vi "Sweep_bias_voltage_GSM-20H10_TektronixMDO.vi"() -> ()   [LabVIEW 2016]
uses:
  <vilib>/Utility/file.llb/Write Delimited Spreadsheet (DBL).vi
panel:
  out "Running index":i32
  out "appended array":sgl[][](array[numeric])
  out "Waveform Graph":sgl[][](graph)
  in  "Number of Points (5)":u32=5
  in  "File Name":string="C:\\Users\\user01\\Desktop\\hsinyeh\\SNSPD_Data\\20230411\\2.5M_6.1K_10photons_0.68uW_"
  out "path":path
  in  "Input voltage":dbl[](array[numeric])
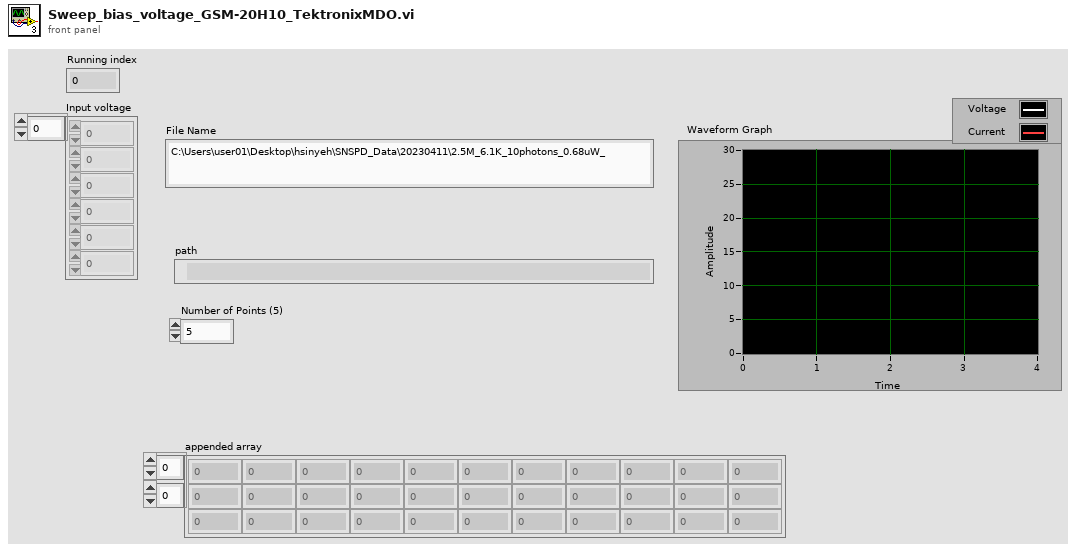
[diagram p1: front panel]
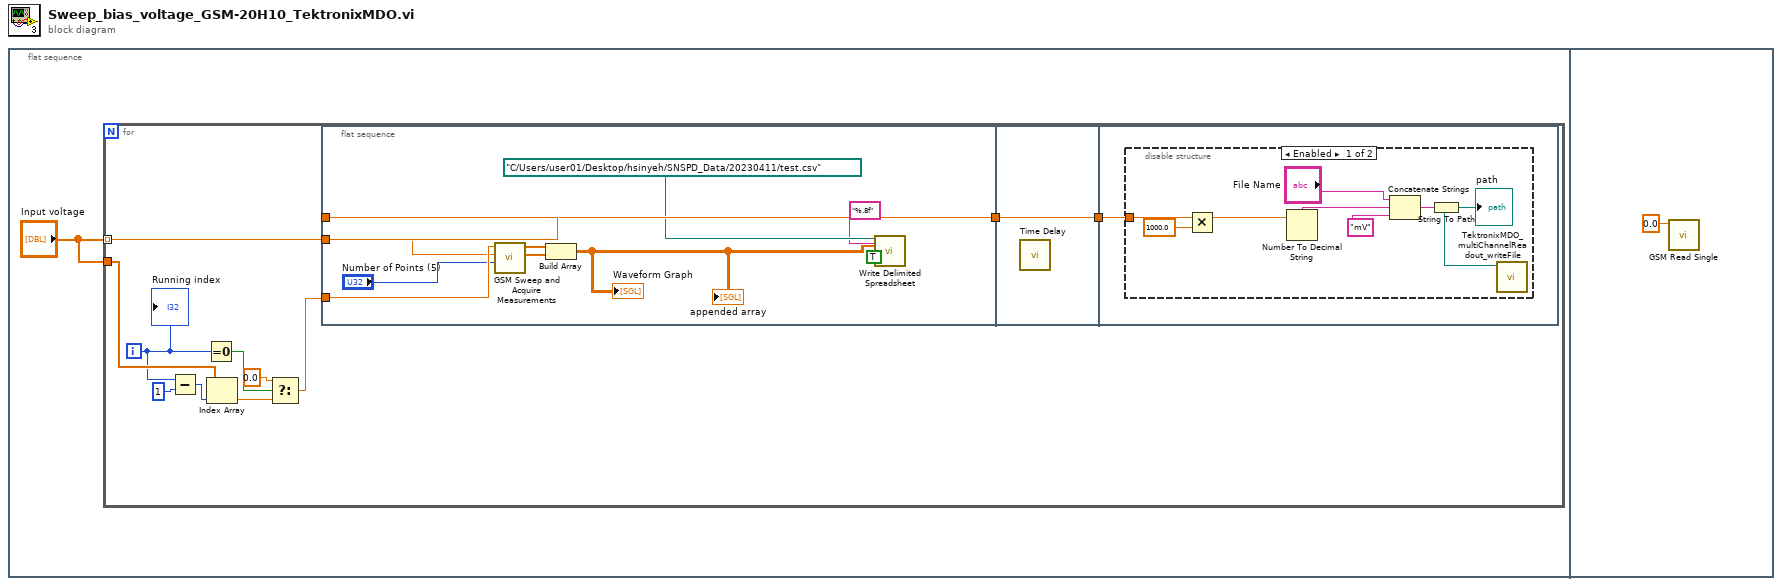
[diagram p0: block diagram]
diagram:
  n1 = flat-sequence {
    frame #0 {
      n2 = for {
        tunnel: "Input voltage" -> [w12] mode=indexing
        tunnel: "Input voltage" -> [w7]
        i -> [w5]
        n3 = Subtract(x=w5, y=1) -> (x-y=w8:i32)
        n4 = Equal To 0?(x=w5) -> (x = 0?=w4:bool)
        n5 = Index Array(array=w7, index=w8) -> (element=w3:dbl)
        n6 = Select(t=0.0, s=w4, f=w3) -> (s? t:f=w2:dbl)
        n7 = flat-sequence {
          tunnel: w12 -> [w17]
          tunnel: w12 -> [w22]
          tunnel: [w22] -> w11
          tunnel: w2 -> [w18]
          tunnel: w11 -> [w23]
          tunnel: [w23] -> w10
          tunnel: w10 -> [w24]
          frame #0 {
            n8 = call <instrlib>:"GSM Sweep and Acquire Measurements.vi"("Number of Points (5)"="Number of Points (5)", "Maximum Amplitude (2)"=w17, "Minimum Amplitude (1)"=w18) -> ("Current"=w14:sgl[], "Voltage"=w15:sgl[])  [unwired: 4 in, 1 out]
            n9 = Build Array(w15, w14) -> (w13:sgl[][])
            "Waveform Graph" <- w13
            "appended array" <- w13
            n10 = call-poly <vilib>:"Write Delimited Spreadsheet.vi"("file path (dialog if empty)"=path "C:/Users/user01/Desktop/hsinyeh/SNSPD_Data/20230411/test.csv", "format (%.3f)"="%.8f", "2D data"=w13, "append to file? (new file:F)"=TRUE) -> ()  [unwired: 10 in, 2 out]
          }
          frame #1 {
            n11 = call "Time Delay"() -> ()  [unwired: 11 in, 1 out]
          }
          frame #2 {
            n12 = disable-structure shown="Enabled" {
              disable-tunnel: w24 -> [w28 _]
              frame Enabled {
                n13 = Multiply(x=w28, y=1000.0) -> (x*y=w26:dbl)
                n14 = Number To Decimal String(number=w26) -> (decimal integer string=w31:string)  [unwired: 1 in]
                n15 = Concatenate Strings("File Name", w31, "mV" ("string")) -> (w29:string)
                n16 = String To Path(string=w29) -> (path=w25:path)
                "path" <- w25
                n17 = call "TektronixMDO_multiChannelReadout_writeFile.vi"("file path"=w25) -> ()  [unwired: 11 in]
              }
              frame Disabled {
              }
            }
          }
        }
        "Running index" <- w5
      }
    }
    frame #1 {
      n18 = call <instrlib>:"GSM Read Single.vi"("Output Level (0)"=0.0) -> ()  [unwired: 8 in, 3 out]
    }
  }
